vi "solar_write ThisLogIgnore.vi"(8 "error in (no error)":errorcluster, 10 "LogIgnore":string[](array[string]), 11 "solar in":refnum<class "solar.lvclass">) -> (0 "error out":errorcluster, 3 "solar out":refnum<class "solar.lvclass">)   [LabVIEW 2018, in "solar.lvclass"]
doc: "This sets the messages to ignore while logging. This is useful to avoid uneccessary entries in the SOLAR logs. Use wildcards as astricks ('*'). Messages are case insensitive.\n - 'MyCMD*' - ignores all messages that start with 'MyCMD'\n - '*' - ignores all commands"
uses:
  solar.lvclass
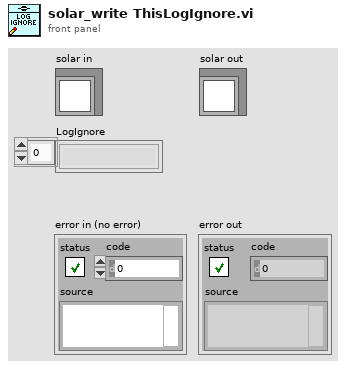
[diagram p1: front panel]
types:
  T1 = typedef "solar_ctl SOLAR Refnum.ctl" = refnum<k1>
  T2 = typedef "solar_ctl SOLAR Global.ctl" = cluster{"Targets":T3[], "AppDir":path, "solar.ini":path, "ConfigsDir":path, "CosmosDir":path, "LogsDir":path, "ExePath":path, "ExeVersion":string, "PartNum":string, "AppSetup":string, "Title":string, "Main.ini":path, "Temp.ini":path, "vSOLAR":string, "Splash.png":string, "SplashWait":i32, "SOLARUE":refnum<user-event>, "VoyagerRefnum":T4, "QTimerRefnum":T5}
  T3 = typedef "solar_ctl Target Global.ctl" = cluster{"Target":string, "Q":refnum<queue>, "UE":refnum<user-event>, "VI":refnum<vi>, "Menu":refnum<k9>, "Data":refnum<data-value>, "Attributes":variant}
  T4 = typedef "solar_voy_ctl Voyager Refnum.ctl" = refnum<k1>
  T5 = typedef "solar_qtimer_ctl Refnum.ctl" = refnum<k1>
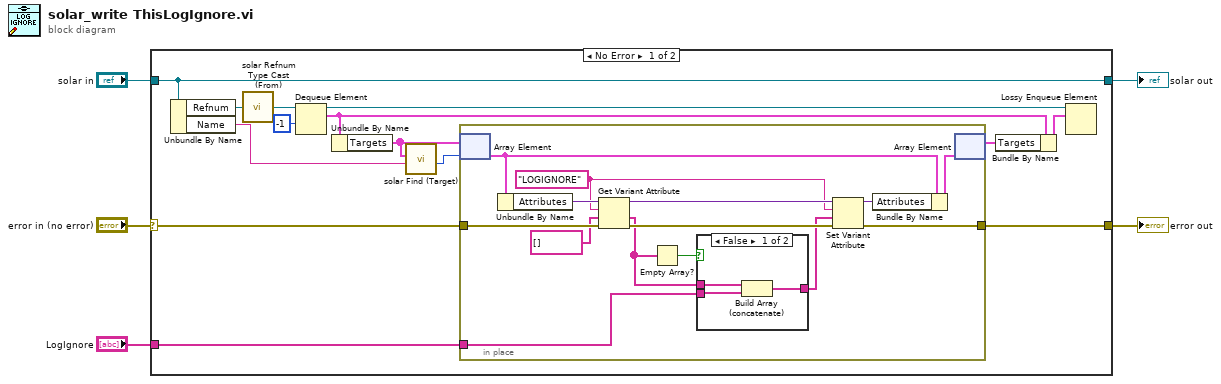
[diagram p0: block diagram]
diagram:
  n1 = case shown="No Error" "error in (no error)" {
    selector: "error in (no error)" -> [w18 w39]
    tunnel: "solar in" -> [w19 w38]
    tunnel: [w15 w39] -> w4
    tunnel: [w19 w38] -> w5
    tunnel: "LogIgnore" -> [w6 _]
    frame No Error {
      n2 = Unbundle By Name(w19) -> ("Refnum"=w17:T1, "Name"=w14:string)
      n3 = call "solar Refnum Type Cast (From).vi"("Refnum"=w17) -> ("SOLAR"=w16:refnum<queue>)
      n4 = Dequeue Element(queue=w16, timeout in ms (-1)=-1) -> (queue out=w13:refnum<queue>, element=w11:T2)  [unwired: 1 in, 2 out]
      n5 = Unbundle By Name(w11) -> ("Targets"=w7:T3[])
      n6 = call "solar Find (Target).vi"("Target"=w14, "Targets"=w7) -> ("Target Index"=w9:i32)  [unwired: 8 in, 1 out]
      n7 = in-place {
        in-place-border: w18 -> [w28]
        in-place-border: [w30] -> w15
        in-place-border: w6 -> [w24]
        w25 = "LOGIGNORE" ("name")
        n8 = in-place-array #1(w7, w9) -> (w33:T3)
        n9 = Unbundle By Name(w33) -> ("Attributes"=w27:variant)
        n10 = Get Variant Attribute(Variant=w27, name=w25, default value (empty Variant)=string[] [], error in=w28) -> (duplicate Variant=w26:variant, value=w20:string[], error out=w29:errorcluster)  [unwired: 1 out]
        n11 = Empty Array?(array=w20) -> (empty?=w21:bool)
        n12 = case shown="False" w21 {
          tunnel: w24 -> [w36 w37]
          tunnel: [w35 w37] -> w23
          tunnel: w20 -> [w34 _]
          frame False {
            n13 = Build Array (concatenate)(w34, w36) -> (w35:string[])
          }
          frame True {
          }
        }
        n14 = Set Variant Attribute(Variant=w26, name=w25, value=w23, error in=w29) -> (Variant out=w31:variant, error out=w30:errorcluster)  [unwired: 1 out]
        n15 = Bundle By Name(cluster=w33, "Attributes"=w31) -> (w32:T3)
        n16 = in-place-array #1(w32) -> (w8:T3[])  [unwired: 1 out]
      }
      n17 = Bundle By Name(cluster=w11, "Targets"=w8) -> (w10:T2)
      n18 = Lossy Enqueue Element(queue=w13, element=w10) -> ()  [unwired: 1 in, 4 out]
    }
    frame Error {
    }
  }
  "error out" <- w4
  "solar out" <- w5
